vi "Convert DBL to string.vi"(9 "Format (%f)":string="%f", 11 "DBL Value":dbl) -> (3 "Converted to String":string)   [LabVIEW 2017, in "XGrapher.xctl"]
uses:
  XGrapher.xctl
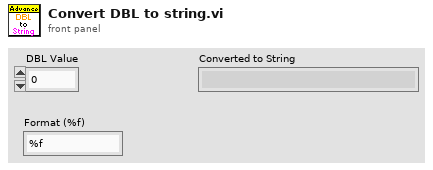
[diagram p1: front panel]
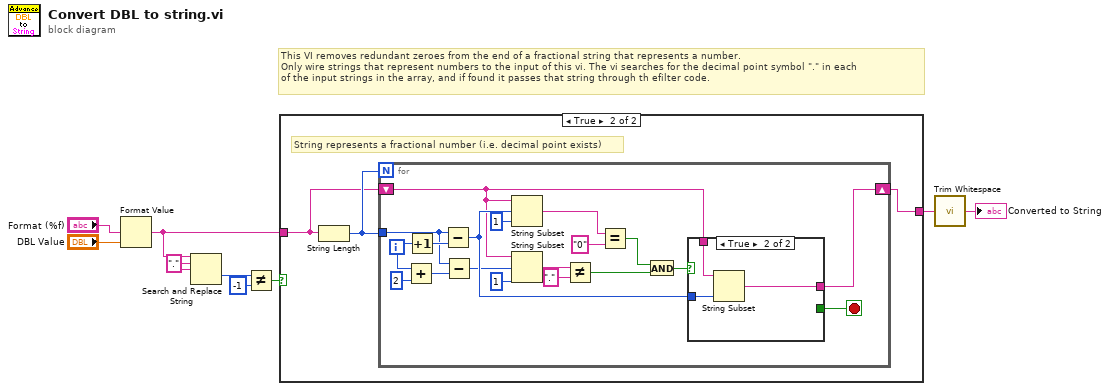
[diagram p0: block diagram]
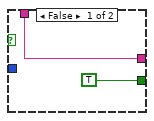
[diagram p3: hidden frame]
diagram:
  w7 = "." ("search string")
  # "This VI removes redundant zeroes from the end of a fractional string that represents a number.\nOnly wire strings that represent numbers to the input of this vi. The vi searches for the decimal point symbol \".\" in each \nof the input strings in the array, and if found it passes that string through th efilter code."
  n1 = Format Value(format string="Format (%f)", value (0)="DBL Value") -> (output string=w3:string)  [unwired: 1 in]
  n2 = Search and Replace String(input string=w3, search string=w7, replace string=w7) -> (offset past replacement=w6:i32)  [unwired: 5 in, 3 out]
  n3 = Not Equal?(x=w6, y=-1) -> (x != y?=w4:bool)
  n4 = case shown="True" w4 {
    tunnel: w3 -> [w10 w11]
    tunnel: [w10 w12] -> w2
    frame False {
    }
    frame True {
      # "String represents a fractional number (i.e. decimal point exists)"
      n5 = String Length(string=w11) -> (length=w13:i32)
      n6 = for {
        N: w13 -> [_]
        tunnel: w13 -> [w16]
        shift-right: [w18] -> w12
        shift-left: w11 -> [w17]
        i -> [w29]
        stop <- w19 stop-if-true
        n7 = Add(x=w29, y=2) -> (x+y=w15:i32)
        n8 = Increment(x=w29) -> (x+1=w31:i32)
        n9 = Subtract(x=w16, y=w31) -> (x-y=w23:i32)
        n10 = Subtract(x=w16, y=w15) -> (x-y=w14:i32)
        n11 = String Subset(string=w17, offset (0)=w23, length (rest)=1 ("length (rest)")) -> (substring=w25:string)
        n12 = String Subset(string=w17, offset (0)=w14, length (rest)=1 ("length (rest)")) -> (substring=w27:string)
        n13 = Not Equal?(x=w27, y=".") -> (x != y?=w21:bool)
        n14 = Equal?(x=w25, y="0") -> (x = y?=w22:bool)
        n15 = And(x=w22, y=w21) -> (x .and. y?=w20:bool)
        n16 = case shown="True" w20 {
          tunnel: w23 -> [_ w37]
          tunnel: [w33 w36] -> w18
          tunnel: w17 -> [w33 w35]
          tunnel: [TRUE _] -> w19
          frame False {
          }
          frame True {
            n17 = String Subset(string=w35, length (rest)=w37) -> (substring=w36:string)  [unwired: 1 in]
          }
        }
      }
    }
  }
  n18 = call <vilib>:"Trim Whitespace.vi"("string"=w2) -> ("trimmed string"=→"Converted to String":string)  [unwired: 1 in]
